vi "SetGlobalVariable.vi"   [LabVIEW 2020, in "Aerotech.lvlib"]
uses:
  Aerotech.lvlib
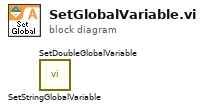
[diagram p0: block diagram]
diagram:
  n1 = call "SetStringGlobalVariable.vi"() -> ()  [unwired: 10 in, 2 out]
  n2 = call "SetDoubleGlobalVariable.vi"() -> ()  [unwired: 10 in, 2 out]
